vi "Sub_Kalman_main.vi"(10 "Experiment":T1, 11 "KF":T2={"State"=[[1.0], [1.0]], "F state prop matrix"=[[1.0, 0.0], [0.0, 1.0]], "H measure matrix"=[[1.0, 0.0]], "P process cov"=[[1.0, 0.0], [0.0, 1.0]], "R measure cov"=[[1.0]], "Q state cov"=[], "T Sample"=0.1, "New Measurement"=10.0, "Measurement Variance"=0.2, "State Variance"=0.2, "Threshold"=0.4, "Initialized"=FALSE}) -> (2 "Experiment":T1, 3 "KF":T2={"State"=[[1.0], [0.0]], "F state prop matrix"=[[1.0, 0.0], [0.0, 1.0]], "H measure matrix"=[[1.0, 0.0]], "P process cov"=[], "R measure cov"=[], "Q state cov"=[], "T Sample"=0.0, "New Measurement"=0.0, "Measurement Variance"=0.0, "State Variance"=0.0, "Threshold"=0.0, "Initialized"=FALSE})   [LabVIEW 2021]
panel:
  out "Waveform Chart 2":dynamicdata(graph)
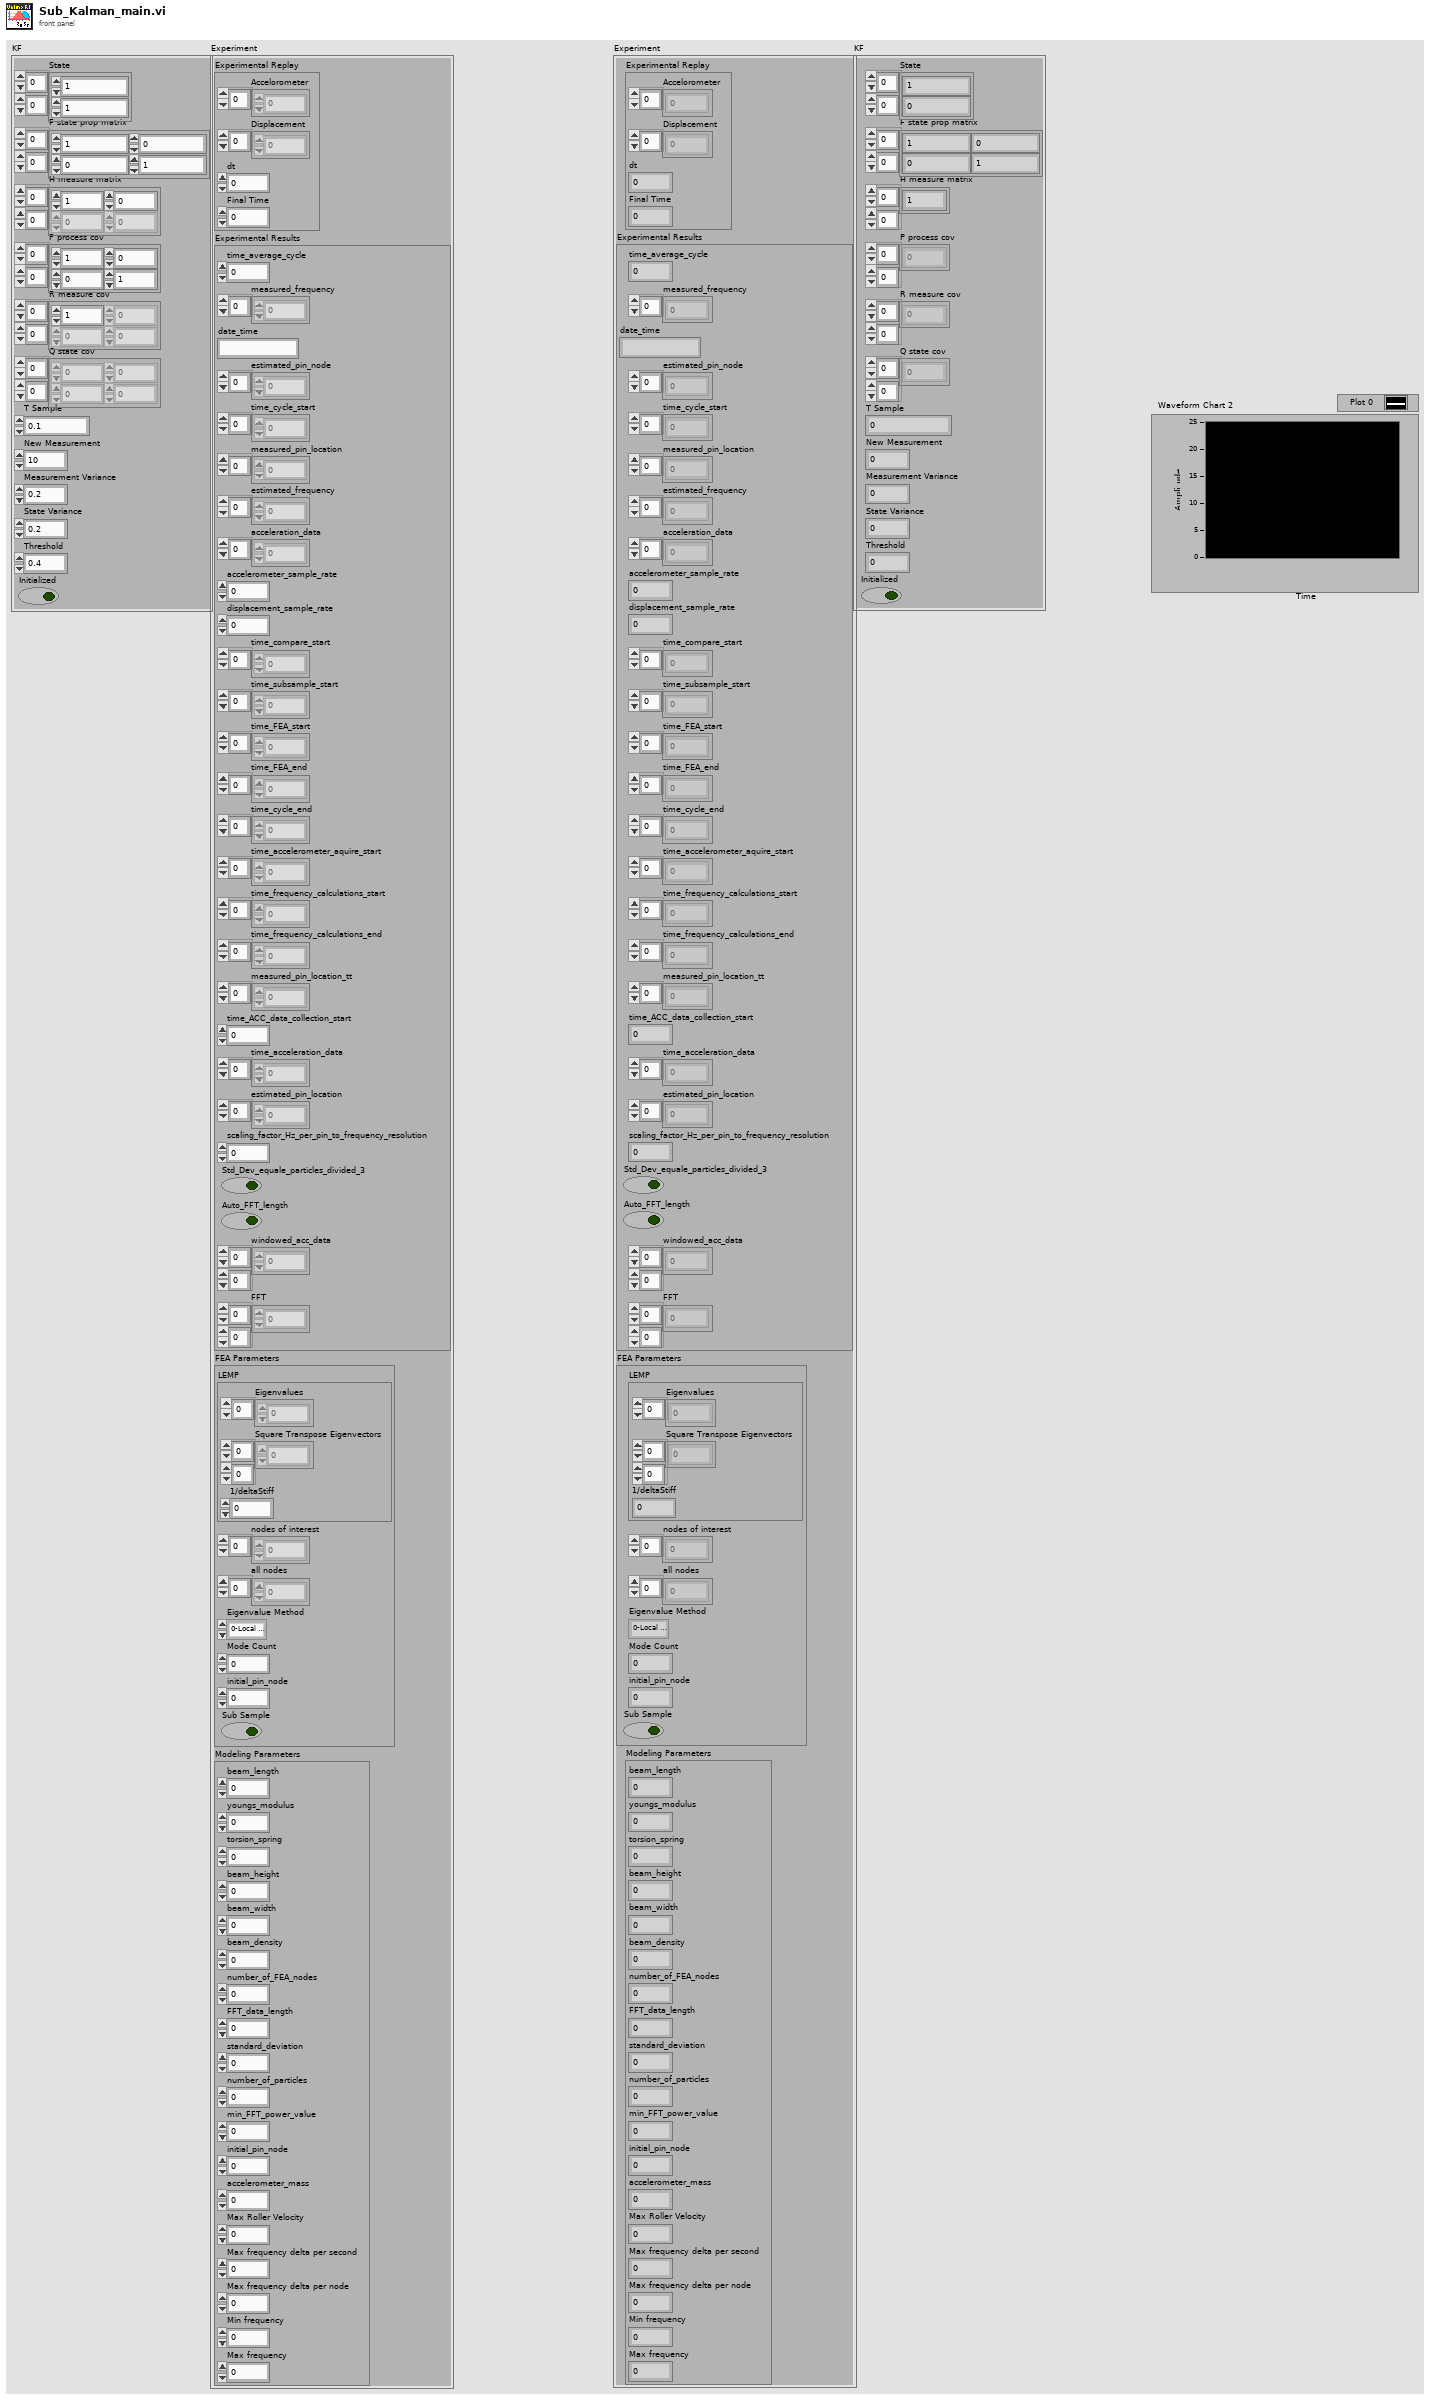
[diagram p1: front panel]
types:
  T1 = cluster{"Experimental Replay":cluster{"Accelorometer":dbl[], "Displacement":dbl[], "dt":dbl, "Final Time":dbl}, "Experimental Results":cluster{"time_average_cycle":dbl, "measured_frequency":dbl[], "date_time":string, "estimated_pin_node":i32[], "time_cycle_start":dbl[], "measured_pin_location":dbl[], "estimated_frequency":dbl[], "acceleration_data":dbl[], "accelerometer_sample_rate":dbl, "displacement_sample_rate":dbl, "time_compare_start":dbl[], "time_subsample_start":dbl[], "time_FEA_start":dbl[], "time_FEA_end":dbl[], "time_cycle_end":dbl[], "time_accelerometer_aquire_start":dbl[], "time_frequency_calculations_start":dbl[], "time_frequency_calculations_end":dbl[], "measured_pin_location_tt":dbl[], "time_ACC_data_collection_start":dbl, "time_acceleration_data":dbl[], "estimated_pin_location":dbl[], "scaling_factor_Hz_per_pin_to_frequency_resolution":dbl, "Std_Dev_equale_particles_divided_3":bool, "Auto_FFT_length":bool, "windowed_acc_data":dbl[][], "FFT":dbl[][]}, "FEA Parameters":cluster{"LEMP":cluster{"Eigenvalues":dbl[], "Square Transpose Eigenvectors":dbl[][], "1/deltaStiff":dbl}, "nodes of interest":i32[], "all nodes":i32[], "Eigenvalue Method":enum16{"0-Local Eigen Modification Procedure", "1-LabVIEW generalized eigenvalues", "2-LabVIEW M^-1K eigenvalues", "3-LabVIEW Cholesky Factorization", "4-Cholesky Factorization CPU SGL", "5-Cholesky Factorization CPU FXP", "6-Cholesky Factorization FPGA SGL", "7-Cholesky Factorization FPGA SGL SCL"}, "Mode Count":i32, "initial_pin_node":i32, "Sub Sample":bool}, "Modeling Parameters":cluster{"beam_length":dbl, "youngs_modulus":dbl, "torsion_spring":dbl, "beam_height":dbl, "beam_width":dbl, "beam_density":dbl, "number_of_FEA_nodes":i32, "FFT_data_length":i32, "standard_deviation":dbl, "number_of_particles":i32, "min_FFT_power_value":dbl, "initial_pin_node":i32, "accelerometer_mass":dbl, "Max Roller Velocity":dbl, "Max frequency delta per second":dbl, "Max frequency delta per node":dbl, "Min frequency":dbl, "Max frequency":dbl}}
  T2 = cluster{"State":dbl[][], "F state prop matrix":dbl[][], "H measure matrix":dbl[][], "P process cov":dbl[][], "R measure cov":dbl[][], "Q state cov":dbl[][], "T Sample":dbl, "New Measurement":dbl, "Measurement Variance":dbl, "State Variance":dbl, "Threshold":dbl, "Initialized":bool}
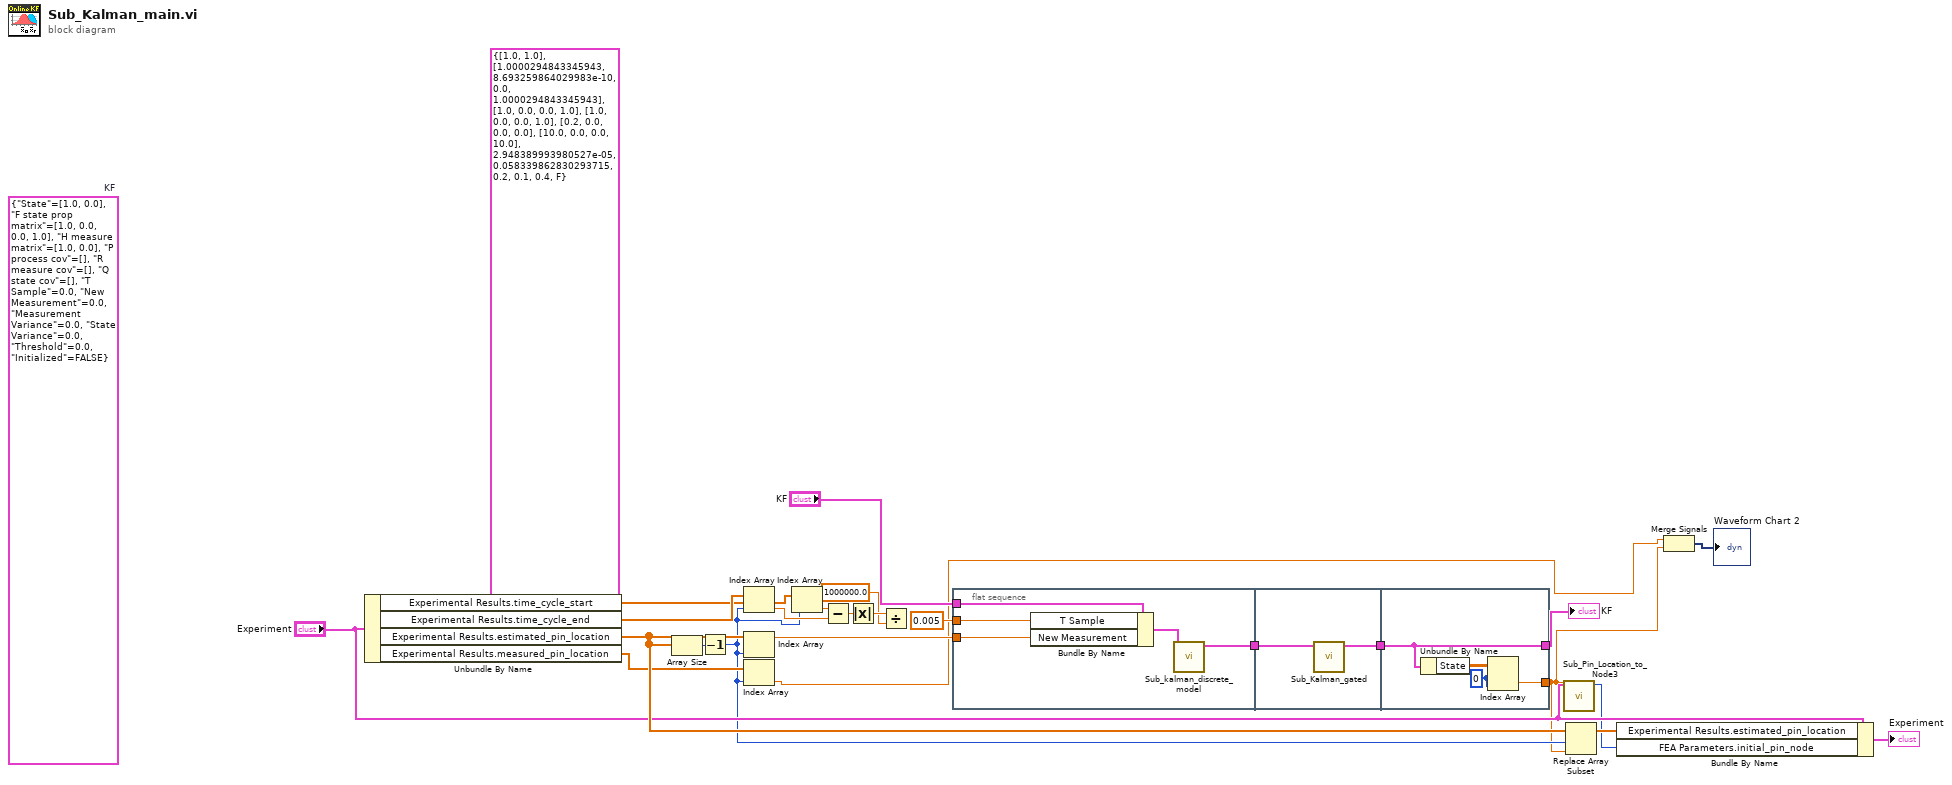
[diagram p0: block diagram]
diagram:
  (unwired) T2 {"State"=[[1.0], [1.0]], "F state prop matrix"=[[1.0000294843345943, 8.693259864029983e-10], [0.0, 1.0000294843345943]], "H measure matrix"=[[1.0, 0.0], [0.0, 1.0]], "P process cov"=[[1.0, 0.0], [0.0, 1.0]], "R measure cov"=[[0.2, 0.0], [0.0, 0.0]], "Q state cov"=[[10.0, 0.0], [0.0, 10.0]], "T Sample"=2.948389993980527e-05, "New Measurement"=0.058339862830293715, "Measurement Variance"=0.2, "State Variance"=0.1, "Threshold"=0.4, "Initialized"=FALSE} ("KF")
  (unwired) T2 {"State"=[[1.0], [0.0]], "F state prop matrix"=[[1.0, 0.0], [0.0, 1.0]], "H measure matrix"=[[1.0, 0.0]], "P process cov"=[], "R measure cov"=[], "Q state cov"=[], "T Sample"=0.0, "New Measurement"=0.0, "Measurement Variance"=0.0, "State Variance"=0.0, "Threshold"=0.0, "Initialized"=FALSE}  # KF
  n1 = Unbundle By Name("Experiment") -> ("Experimental Results.time_cycle_start"=w10:dbl[], "Experimental Results.time_cycle_end"=w15:dbl[], "Experimental Results.estimated_pin_location"=w20:dbl[], "Experimental Results.measured_pin_location"=w6:dbl[])
  n2 = Array Size(array=w20) -> (size(s)=w21:i32)
  n3 = Decrement(x=w21) -> (x-1=w5:i32)
  n4 = Index Array(array=w15, index=w5) -> (element=w13:dbl)
  n5 = Index Array(array=w20, index=w5) -> (element=w7:dbl)
  n6 = Index Array(array=w6, index=w5) -> (element=w3:dbl)
  n7 = Index Array(array=w10, index=w5) -> (element=w14:dbl)
  n8 = Subtract(x=w14, y=w13) -> (x-y=w12:dbl)
  n9 = Absolute Value(x=w12) -> (abs(x)=w9:dbl)
  n10 = Divide(x=w9, y=1000000.0) -> ()  [unwired: 1 out]
  n11 = flat-sequence {
    tunnel: [w28] -> w24
    tunnel: 0.005 -> [w27]
    tunnel: "KF" -> [w26]
    tunnel: w7 -> [w25]
    tunnel: w24 -> [w31]
    tunnel: [w30] -> w22
    tunnel: [w34] -> w23
    tunnel: w22 -> [w34]
    tunnel: [w32] -> w2
    frame #0 {
      n12 = Bundle By Name(cluster=w26, "T Sample"=w27, "New Measurement"=w25) -> (w29:T2)
      n13 = call "Sub_kalman_discrete_model.vi"("KF"=w29) -> ("KF"=w28:T2)  [unwired: 10 in]
    }
    frame #1 {
      n14 = call "Sub_Kalman_gated.vi"("KF"=w31) -> ("KF"=w30:T2)  [unwired: 10 in]
    }
    frame #2 {
      w33 = 0 ("index (row)")
      n15 = Unbundle By Name(w34) -> ("State"=w35:dbl[][])
      n16 = Index Array(array=w35, index (row)=w33, index (col)=w33) -> (element=w32:dbl)
    }
  }
  n17 = call "Sub_Pin_Location_to_Node3.vi"("Pin Location"=w2, "Experiment in"="Experiment") -> ("DOF of Interest"=w16:i32)  [unwired: 9 in]
  n18 = Replace Array Subset(array=w20, new element=w2, index=w5) -> (w19:dbl[])
  n19 = Bundle By Name(cluster="Experiment", "Experimental Results.estimated_pin_location"=w19, "FEA Parameters.initial_pin_node"=w16) -> (→"Experiment":T1)
  n20 = Merge Signals(w3, w2) -> (→"Waveform Chart 2":dynamicdata)
  "KF" <- w23
